vi "Load Classes.vi"(8 "error in (no error)":errorcluster, 10 "class paths":path[](array[path]), 11 "Component Loader in":refnum<class "Component Loader.lvclass">) -> (0 "error out":errorcluster, 2 "objects":refnum<class>[](array[class]), 3 "Component Loader out":refnum<class "Component Loader.lvclass">)   [LabVIEW 2017, in "Data Sharing Framework Core.lvlib" / "Data Sharing Framework Engine.lvlib" / "Component Loader.lvclass"]
uses:
  Component Loader.lvclass
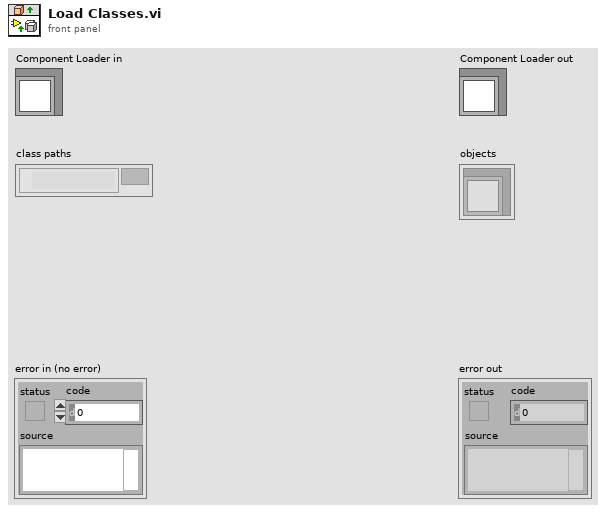
[diagram p1: front panel]
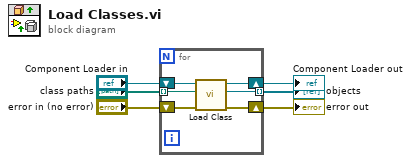
[diagram p0: block diagram]
diagram:
  n1 = for {
    tunnel: [w12] -> w5 mode=indexing
    shift-right: [w11] -> w3
    shift-left: "Component Loader in" -> [w10]
    tunnel: "class paths" -> [w9] mode=indexing
    shift-right: [w8] -> w2
    shift-left: "error in (no error)" -> [w7]
    n2 = call "Load Class.vi"("error in (no error)"=w7, "class path"=w9, "Component Loader in"=w10) -> ("error out"=w8:errorcluster, "object"=w12:refnum<class>, "Component Loader out"=w11:refnum<class "Component Loader.lvclass">)  [unwired: 6 in]
  }
  "error out" <- w2
  "Component Loader out" <- w3
  "objects" <- w5
